vi "CT path.vi"(11 "path":path) -> (1 "path 1":path, 2 "file exists?":bool, 3 "path 2":path)   [LabVIEW 2016]
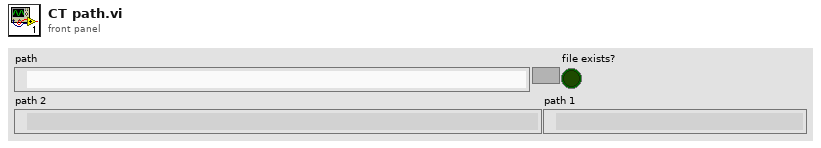
[diagram p1: front panel]
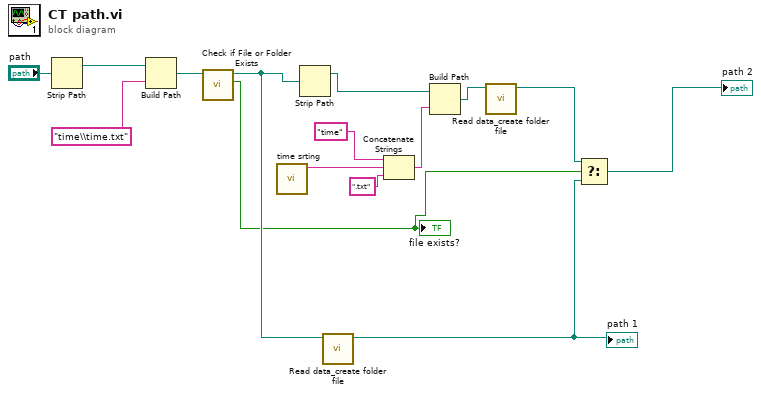
[diagram p0: block diagram]
diagram:
  n1 = Strip Path(path="path") -> (stripped path=w14:path)  [unwired: 1 out]
  n2 = Build Path(base path=w14, name or relative path="time\\time.txt") -> (appended path=w13:path)
  n3 = call <vilib>:"Check if File or Folder Exists.vi"("path"=w13) -> ("file or folder exists?"=w3:bool, "dup path"=w5:path)  [unwired: 8 in, 1 out]
  "file exists?" <- w3
  n4 = call "time srting.vi"() -> ("date/time string"=w11:string)  [unwired: 11 in]
  n5 = Strip Path(path=w5) -> (stripped path=w9:path)  [unwired: 1 out]
  n6 = call "Read data_create folder file.vi"("path"=w5) -> ("dup path"=w1:path)  [unwired: 10 in]
  "path 1" <- w1
  n7 = Concatenate Strings("time" ("string"), w11, ".txt" ("string")) -> (w10:string)
  n8 = Build Path(base path=w9, name or relative path=w10) -> (appended path=w7:path)
  n9 = call "Read data_create folder file.vi"("path"=w7) -> ("dup path"=w4:path)  [unwired: 10 in]
  n10 = Select(t=w4, s=w3, f=w1) -> (s? t:f=→"path 2":path)
